vi "external_trigger_demo.vi"() -> ()   [LabVIEW 2012]
uses:
  <vilib>/DAQmx/write.llb/DAQmx Write (Digital Bool 1Line 1Point).vi
  <vilib>/DAQmx/create/channels.llb/DAQmx Create Channel (DO-Digital Output).vi
  <vilib>/DAQmx/miscellaneous.llb/DAQmx Fill In Error Info.vi
panel:
  out "DevInq1":errorcluster
  in  "Stop Movie":bool
  in  "Trigger T/F":bool
  in  "DMD_trigger":tag="Dev1/port0/line7" caption="DMD trigger"
  out "Error out":errorcluster
  in  "Error in (no error)":errorcluster
  in  "SequenceRepeats":i32=1
  in  "binary mov path":path=path "C:/Users/cohen_lab/Desktop/Labview_code/DMD_control/DMD6images.bin"
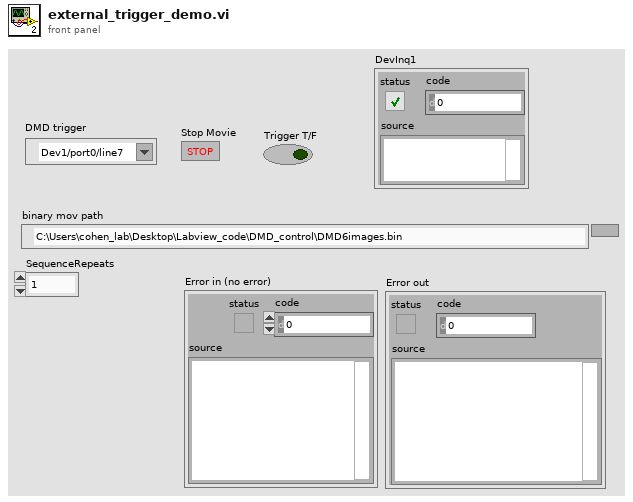
[diagram p1: front panel]
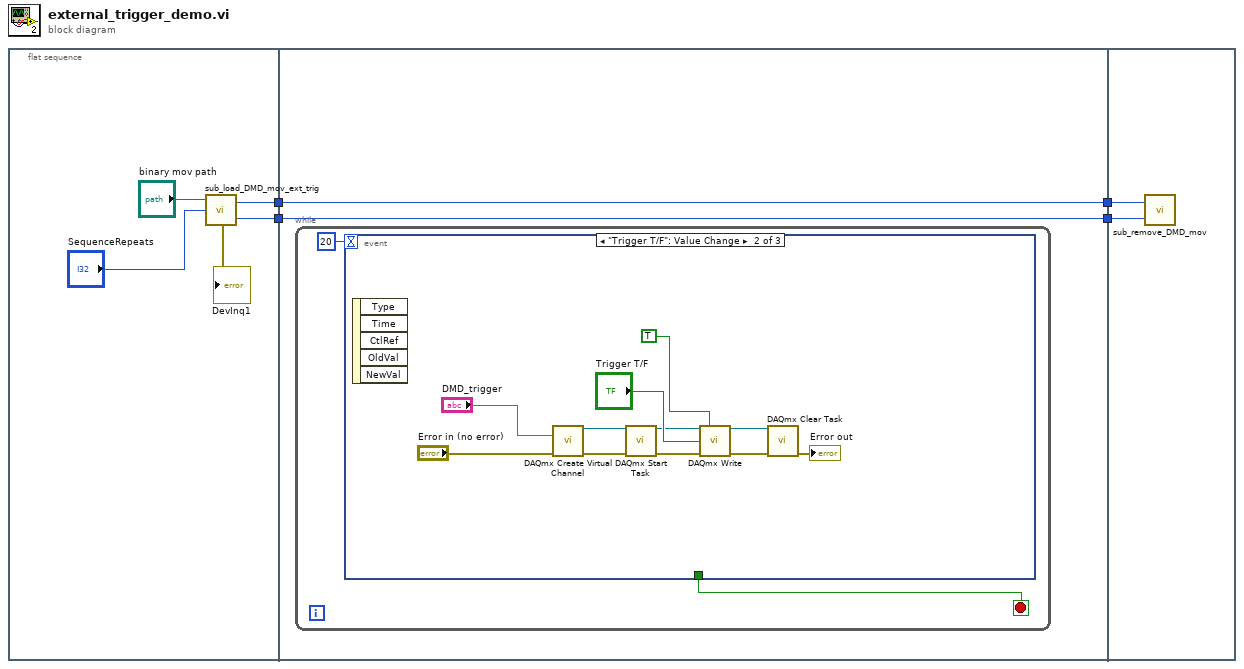
[diagram p0: block diagram]
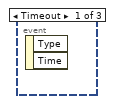
[diagram p2: hidden frame]
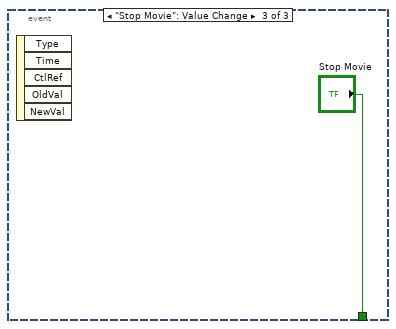
[diagram p3: hidden frame]
diagram:
  n1 = flat-sequence {
    tunnel: [w7] -> w3
    tunnel: [w6] -> w1
    tunnel: [w11] -> w4
    tunnel: w3 -> [w11]
    tunnel: [w10] -> w2
    tunnel: w1 -> [w10]
    tunnel: w4 -> [w27]
    tunnel: w2 -> [w26]
    frame #0 {
      n2 = call "sub_load_DMD_mov_ext_trig.vi"("SequenceRepeats"="SequenceRepeats", "binary mov path"="binary mov path") -> ("SequID"=w6:u32, "DeviceID"=w7:u32, "DevInq1"=→"DevInq1":errorcluster)
    }
    frame #1 {
      n3 = while {
        stop <- w13 stop-if-true
        n4 = event shown="[1] \"Trigger T/F\": Value Change" {
          selector: _ -> [_ _ _]
          dyn-events: _ -> [_ _ _]
          timeout: 20 -> [_ _ _]
          tunnel: [_ _ "Stop Movie"] -> w13
          event Timeout {
            n5 = event-data() -> ()  [unwired: 1 in, 2 out]
          }
          event "Trigger T/F": Value Change {
            n6 = event-data() -> ()  [unwired: 1 in, 5 out]
            n7 = call-poly <vilib>:"DAQmx Create Virtual Channel.vi"("lines"="DMD_trigger", "error in"="Error in (no error)") -> ("task out"=w20:refnum<k21>, "error out"=w19:errorcluster)  [unwired: 3 in, 9 out]
            n8 = call <vilib>:"DAQmx Start Task.vi"("task/channels in"=w20, "error in"=w19) -> ("task out"=w17:refnum<k21>, "error out"=w14:errorcluster)  [unwired: 12 out]
            n9 = call-poly <vilib>:"DAQmx Write.vi"("task/channels in"=w17, "auto start"=TRUE, "data"="Trigger T/F", "error in"=w14) -> ("task out"=w16:refnum<k21>, "error out"=w15:errorcluster)  [unwired: 9 in, 1 out]
            n10 = call <vilib>:"DAQmx Clear Task.vi"("task in"=w16, "error in"=w15) -> ("error out"=→"Error out":errorcluster)  [unwired: 13 out]
          }
          event "Stop Movie": Value Change {
            n11 = event-data() -> ()  [unwired: 1 in, 5 out]
          }
        }
      }
    }
    frame #2 {
      n12 = call "sub_remove_DMD_mov.vi"("SequenceId"=w26, "DeviceId"=w27) -> ()  [unwired: 2 out]
    }
  }
